vi "Read Names.vi"(8 "error in (no error)":errorcluster, 11 "DAC ADV in":refnum<class "DAC ADV.lvclass">) -> (0 "error out":errorcluster, 2 "Names":string="Vx,Vy,Vz,A1,A2,A3,C1,C2,C3", 3 "DAC ADV out":refnum<class "DAC ADV.lvclass">)   [LabVIEW 2019, in "DAC.lvlib" / "DAC ADV.lvclass"]
uses:
  DAC ADV.lvclass
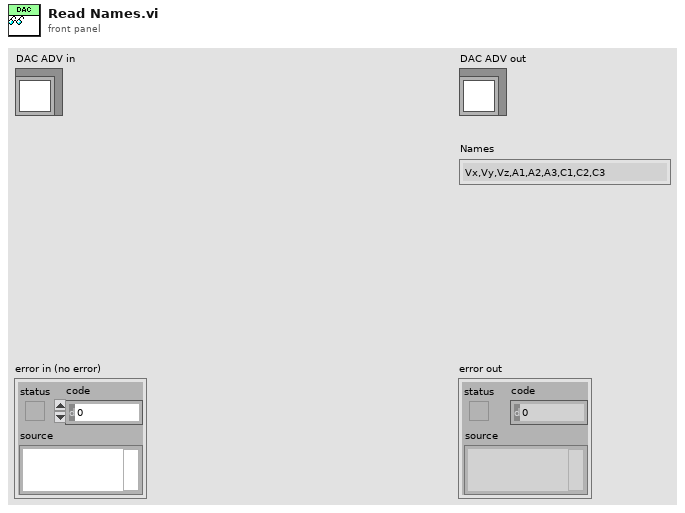
[diagram p1: front panel]
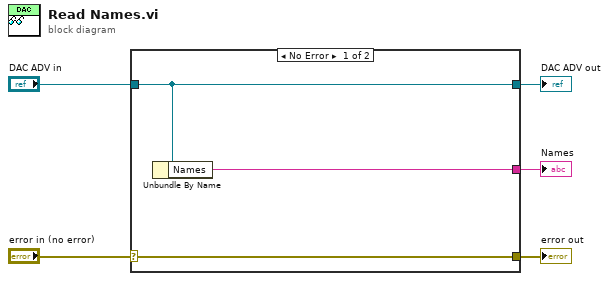
[diagram p0: block diagram]
diagram:
  n1 = case shown="No Error" "error in (no error)" {
    selector: "error in (no error)" -> [w8 w9]
    tunnel: [w8 w9] -> w4
    tunnel: [w7 w10] -> w2
    tunnel: "DAC ADV in" -> [w7 w10]
    tunnel: [w6 _] -> w1
    frame No Error {
      n2 = Unbundle By Name(w7) -> ("Names"=w6:string)
    }
    frame Error {
    }
  }
  "error out" <- w4
  "DAC ADV out" <- w2
  "Names" <- w1
